vi "SaveFile.vi"(6 "TyprControl":bool, 8 "error in (no error)":errorcluster, 9 "text":string, 10 "file path (use dialog)":path, 11 "XuLyDataDisplay in":refnum<class "XuLyDataDisplay.lvclass">) -> (0 "error out":errorcluster, 3 "XuLyDataDisplay out":refnum<class "XuLyDataDisplay.lvclass">)   [LabVIEW 2017, in "LibraryGcode.lvlib" / "XuLyDataDisplay.lvclass"]
uses:
  XuLyDataDisplay.lvclass
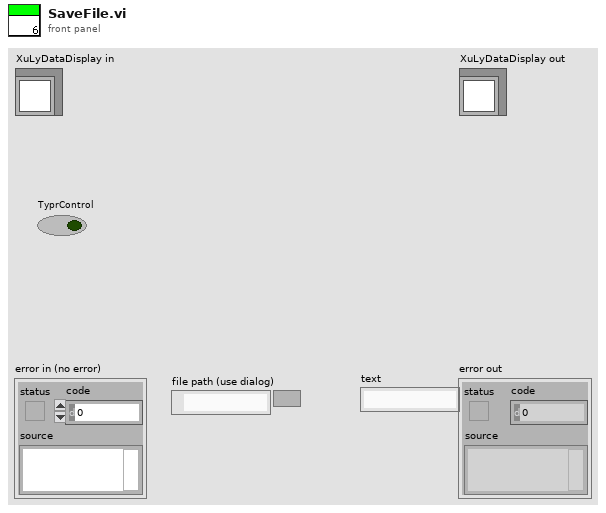
[diagram p1: front panel]
types:
  T1 = enum16{"open", "replace", "create", "open or create", "replace or create", "replace or create with confirmation"}
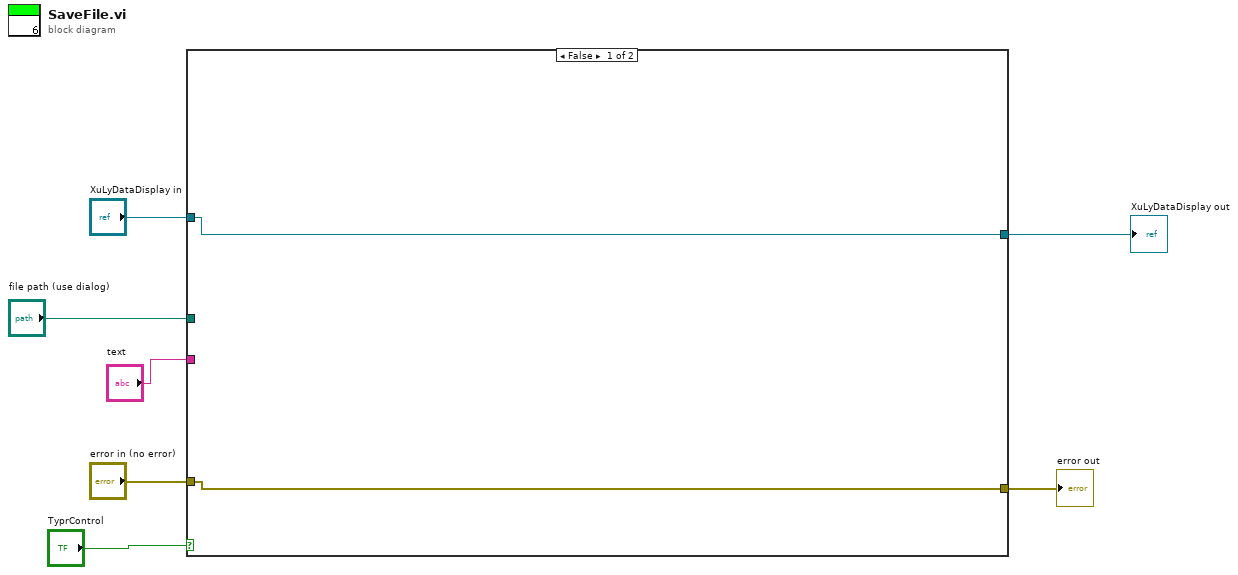
[diagram p0: block diagram]
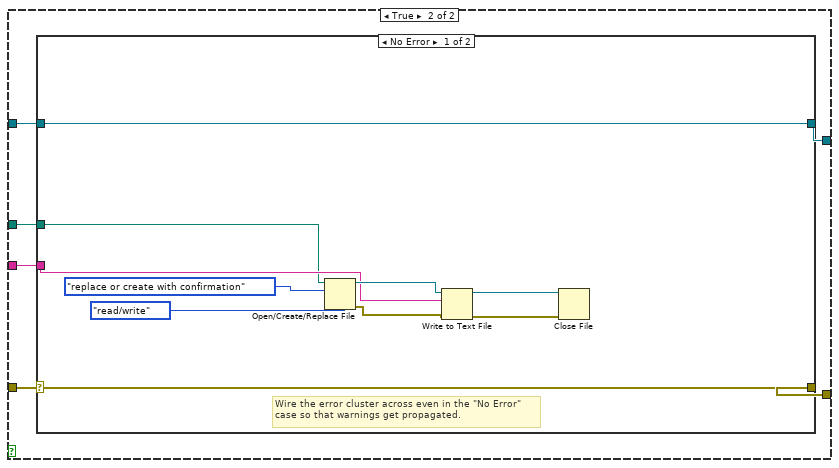
[diagram p2: hidden frame]
diagram:
  n1 = case shown="False" "TyprControl" {
    tunnel: "error in (no error)" -> [w8 w15]
    tunnel: [w8 w14] -> w6
    tunnel: "XuLyDataDisplay in" -> [w9 w13]
    tunnel: [w9 w12] -> w4
    tunnel: "text" -> [_ w11]
    tunnel: "file path (use dialog)" -> [_ w10]
    frame False {
    }
    frame True {
      n2 = case shown="No Error" w15 {
        selector: w15 -> [w24 w27]
        tunnel: [w24 w27] -> w14
        tunnel: [w25 w26] -> w12
        tunnel: w13 -> [w25 w26]
        tunnel: w11 -> [w17 _]
        tunnel: w10 -> [w16 _]
        frame No Error {
          # "Wire the error cluster across even in the \"No Error\"\ncase so that warnings get propagated."
          n3 = Open/Create/Replace File(file path (use dialog)=w16, operation (0:open)=T1."replace or create with confirmation", access (0:read/write)=enum16{"read/write", "read-only", "write-only"}."read/write") -> (refnum out=w18:refnum<file>, error out=w21:errorcluster)  [unwired: 3 in, 1 out]
          n4 = Write to Text File(file (use dialog)=w18, text=w17, error in=w21) -> (refnum out=w19:refnum<file>, error out=w20:errorcluster)  [unwired: 1 in, 1 out]
          n5 = Close File(refnum=w19, error in=w20) -> ()  [unwired: 2 out]
        }
        frame Error {
        }
      }
    }
  }
  "error out" <- w6
  "XuLyDataDisplay out" <- w4
